vi "BenchConfig_Init.vi"(8 "error in (no error)":errorcluster) -> (0 "error out":errorcluster, 3 "BenchConfig":T1)   [LabVIEW 2011]
uses:
  BenchConfig.ctl
panel:
  # "A configurer"
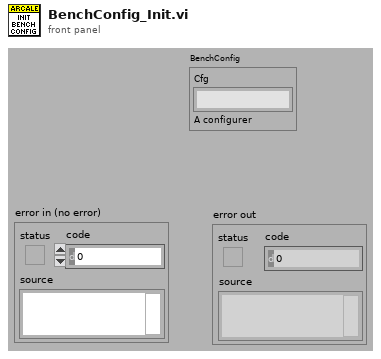
[diagram p1: front panel]
types:
  T1 = typedef "BenchConfig.ctl" = cluster{"Cfg":string}
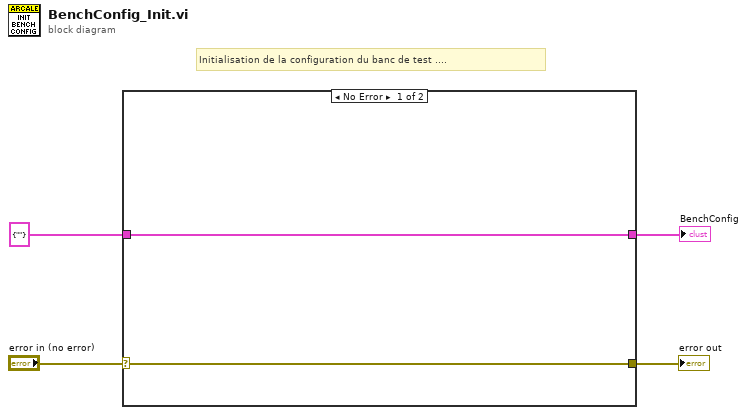
[diagram p0: block diagram]
diagram:
  # "Initialisation de la configuration du banc de test ...."
  n1 = case shown="No Error" "error in (no error)" {
    selector: "error in (no error)" -> [w6 w7]
    tunnel: [w6 w7] -> w3
    tunnel: T1 {"Cfg"=""} ("BenchConfig") -> [w5 w8]
    tunnel: [w5 w8] -> w1
    frame No Error {
    }
    frame Error {
    }
  }
  "error out" <- w3
  "BenchConfig" <- w1
